vi "Draw Crosshair.vi"(8 "error in":errorcluster, 9 "xhair name":string="donotrename", 10 "Crosshair":T1={"Draw"=TRUE, "Target"={"x"=20.0, "y"=20.0}, "Size"={"x"=20.0, "y"=20.0}, "Angle"=1250067.0, "Color"=1250067, "Thickness"=20, "CrosshairLabel"=""} {"Thickness" max=0; "Target"."y" min=0.0 max=0.0; "Target"."x" min=0.0 max=0.0; "Angle" format="%#_13g"; "Size"."y" min=0.0 max=0.0; "Size"."x" min=0.0 max=0.0}, 11 "Image in":T2) -> (0 "error out":errorcluster, 3 "image out":T2)   [LabVIEW 2013]
doc: "Draw Crosshair in image as per targetx and y and size\ninput:\n1. Draw crosshair cluster (Image in, Draw(boolean), size, target x, target y)\n2. Error in\noutput\n1.Error out"
uses:
  <vilib>/vision/Image Controls.llb/IMAQ Image.ctl
  Controls/Crosshair type def.ctl
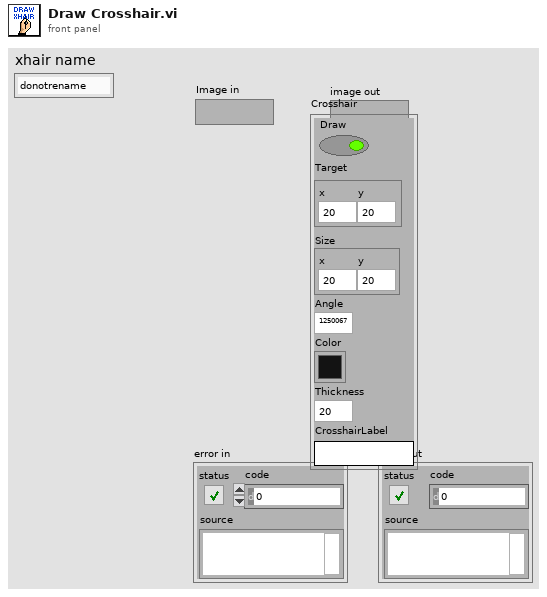
[diagram p1: front panel]
types:
  T1 = typedef "Crosshair type def.ctl" = cluster{"Draw":bool, "Target":cluster{"x":dbl, "y":dbl}, "Size":cluster{"x":dbl, "y":dbl}, "Angle":dbl, "Color":u32, "Thickness":u8, "CrosshairLabel":string}
  T2 = typedef "IMAQ Image.ctl" = refnum<image>
  T3 = cluster{"Left":i32, "Top":i32, "Right":i32, "Bottom":i32}
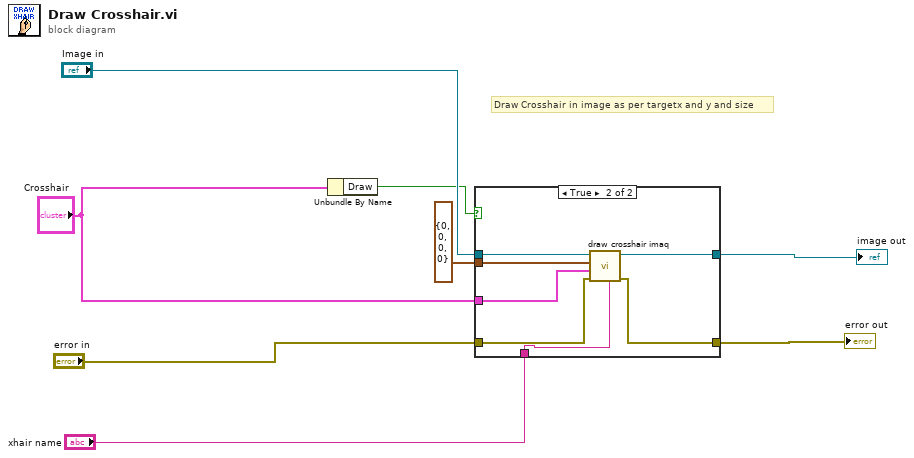
[diagram p0: block diagram]
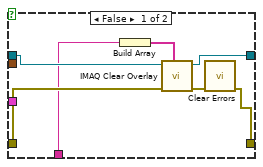
[diagram p2: hidden frame]
diagram:
  # "Draw Crosshair in image as per targetx and y and size"
  n1 = Unbundle By Name("Crosshair") -> ("Draw"=w2:bool)
  n2 = case shown="True" w2 {
    tunnel: "Image in" -> [w15 w22]
    tunnel: [w14 w20] -> w5
    tunnel: T3 {"Left"=0, "Top"=0, "Right"=0, "Bottom"=0} ("Bounding Rectangle") -> [_ w21]
    tunnel: "error in" -> [w11 w19]
    tunnel: [w10 w18] -> w7
    tunnel: "xhair name" -> [w9 w17]
    tunnel: "Crosshair" -> [_ w16]
    frame False {
      n3 = Build Array(w9) -> (w12:string[])
      n4 = call "IMAQ Clear Overlay"("Groups"=w12, "error in (no error)"=w11, "Image"=w15) -> ("error out"=w13:errorcluster, "Image Out"=w14:T2)  [unwired: 7 in]
      n5 = call <vilib>:"Clear Errors.vi"("error in (no error)"=w13) -> ("error out"=w10:errorcluster)  [unwired: 6 in]
    }
    frame True {
      n6 = call "draw crosshair imaq.vi"("overlay name"=w17, "error in (no error)"=w19, "Crosshair"=w16, "Bounding Rectangle"=w21, "image in"=w22) -> ("error out"=w18:errorcluster, "image out"=w20:T2)  [unwired: 5 in]
    }
  }
  "error out" <- w7
  "image out" <- w5
